vi "Read Spectrum.vi"(8 "error in (no error)":errorcluster, 11 "VISA resource name":refnum<visa-resource-name>) -> (0 "error out":errorcluster, 1 "Black Pixel Median":dbl, 2 "Spectrum by Pixel Number":dbl[](array[numeric]), 3 "VISA resource name out":refnum<visa-resource-name>)   [LabVIEW 2012, in "Ocean Optics 2000 4000.lvlib"]
doc: "Reads the optical or full spectra from the spectrometer, based on Pixel Mode selected in <b>Initalize</b> VI. The spectrum is displayed in an array according to the pixel number."
uses:
  Ocean Optics 2000 4000.lvlib
  <vilib>/Analysis/NI_AALBase.lvlib
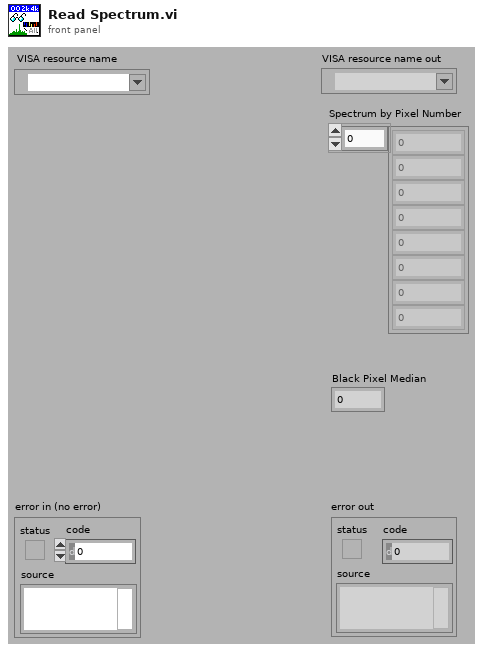
[diagram p1: front panel]
types:
  T1 = cluster{"Start Pixel":i32, "Stop Pixel":i32, "Start Black":i32[], "Stop Black":i32[]}
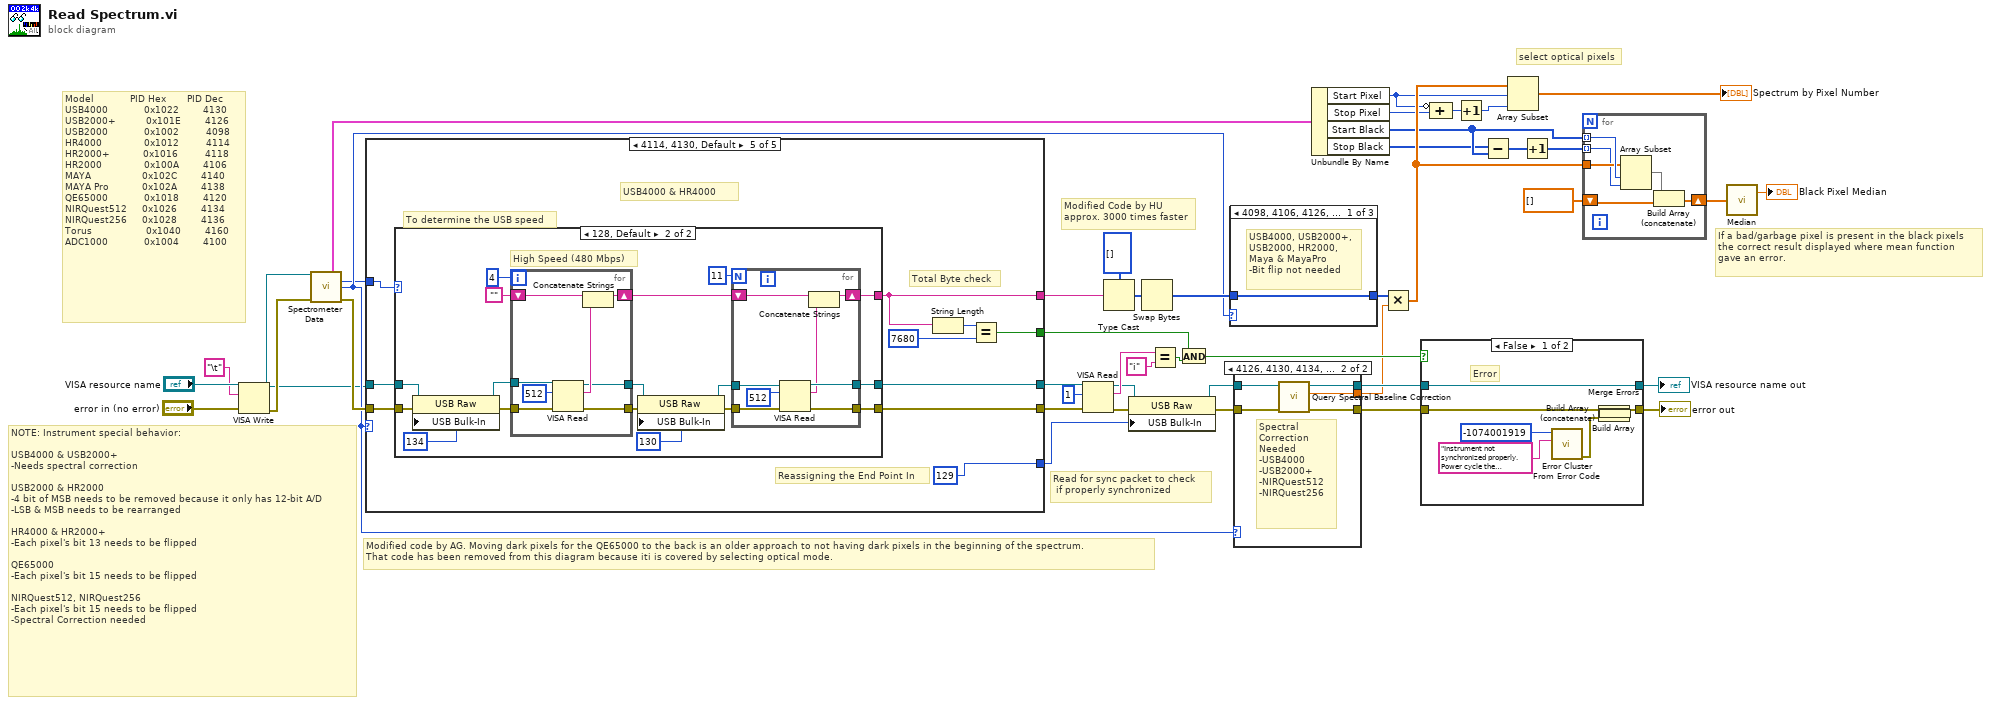
[diagram p0: block diagram]
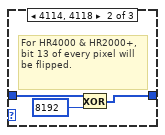
[diagram p2: hidden frame]
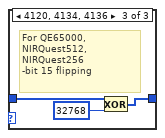
[diagram p3: hidden frame]
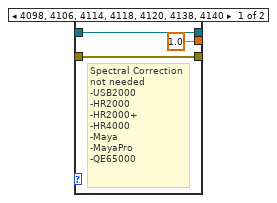
[diagram p4: hidden frame]
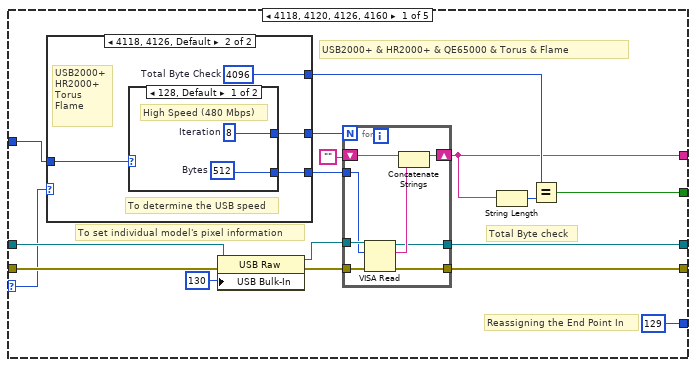
[diagram p5: hidden frame]
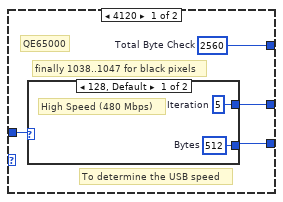
[diagram p6: hidden frame]
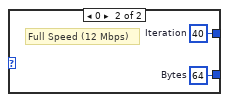
[diagram p7: hidden frame]
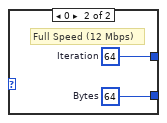
[diagram p8: hidden frame]
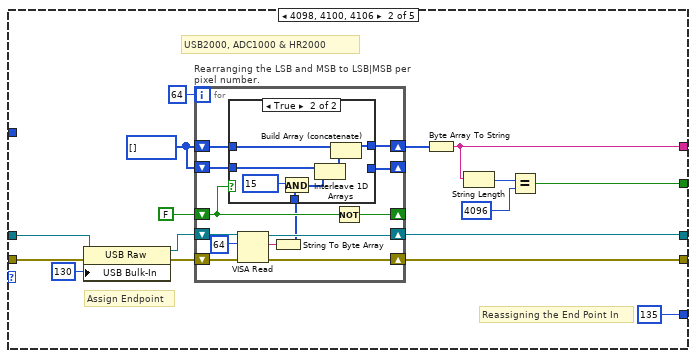
[diagram p9: hidden frame]
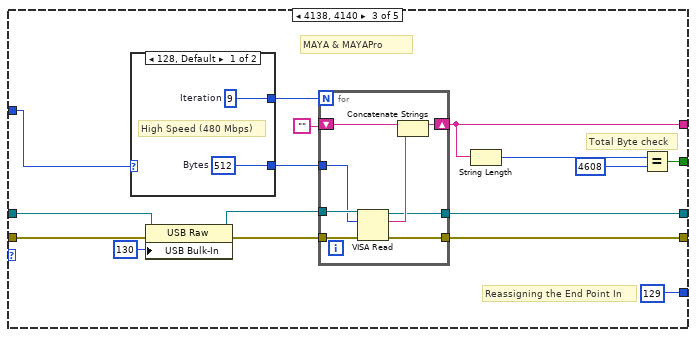
[diagram p11: hidden frame]
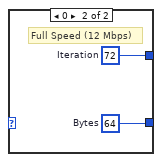
[diagram p12: hidden frame]
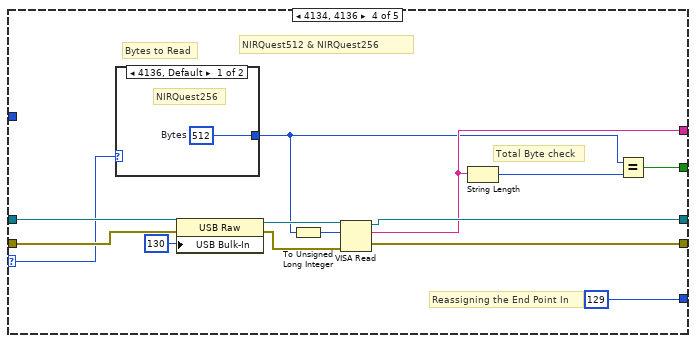
[diagram p13: hidden frame]
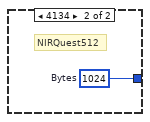
[diagram p14: hidden frame]
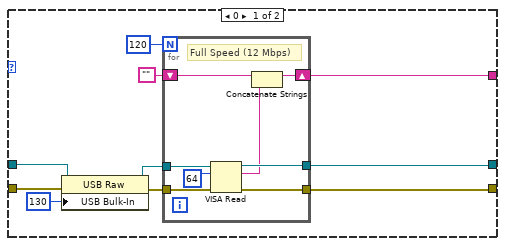
[diagram p15: hidden frame]
diagram:
  # "If a bad/garbage pixel is present in the black pixels\nthe correct result displayed where mean function\ngave an error."
  # "select optical pixels"
  # "Modified code by AG. Moving dark pixels for the QE65000 to the back is an older approach to not having dark pixels in the beginning of the spectrum.\nThat code has been removed from this diagram because iti is covered by selecting optical mode."
  # "Model            PID Hex       PID Dec \nUSB4000            0x1022        4130 \nUSB2000+          0x101E        4126 \nUSB2000            0x1002         4098\nHR4000              0x1012         4114\nHR2000+           0x1016         4118\nHR2000              0x100A        4106\nMAYA                 0x102C        4140\nMAYA Pro           0x102A        4138\nQE65000            0x1018        4120\nNIRQuest512     0x1026        4134\nNIRQuest256     0x1028        4136\nTorus                  0x1040        4160\nADC1000            0x1004        4100"
  # "Modified Code by HU\napprox. 3000 times faster"
  # "NOTE: Instrument special behavior:\n\nUSB4000 & USB2000+ \n-Needs spectral correction\n\nUSB2000 & HR2000\n-4 bit of MSB needs to be removed because it only has 12-bit A/D\n-LSB & MSB needs to be rearranged \n\nHR4000 & HR2000+\n-Each pixel's bit 13 needs to be flipped\n\nQE65000\n-Each pixel's bit 15 needs to be flipped\n\nNIRQuest512, NIRQuest256\n-Each pixel's bit 15 needs to be flipped \n-Spectral Correction needed"
  # "Read for sync packet to check\n if properly synchronized"
  n1 = VISA Write(VISA resource name="VISA resource name", write buffer="\t", error in (no error)="error in (no error)") -> (VISA resource name out=w2:refnum<visa-resource-name>, error out=w4:errorcluster)  [unwired: 1 out]
  n2 = call "Spectrometer Data.vi"("VISA resource name"=w2, "error in (no error)"=w4) -> ("Pixels"=w11:T1, "USB Speed"=w1:u16, "ID"=w3:u16, "error out"=w20:errorcluster)  [unwired: 8 in, 2 out]
  n3 = case shown="4114, 4130, Default" w3 {
    selector: w3 -> [w49 _ _ w161 _]
    tunnel: w2 -> [w61 w101 w140 w163 w178]
    tunnel: w20 -> [w62 w100 w139 w162 w177]
    tunnel: [w47 w89 w127 w156 w171] -> w27
    tunnel: [w60 w88 w138 w158 w176] -> w44
    tunnel: [w59 w87 w137 w157 w175] -> w43
    tunnel: [w58 w97 w134 w159 w173] -> w29
    tunnel: [i16 129 ("USB Settings:Bulk-In Pipe") i16 135 ("USB Settings:Bulk-In Pipe") i16 129 ("USB Settings:Bulk-In Pipe") i16 129 ("USB Settings:Bulk-In Pipe") i16 129 ("USB Settings:Bulk-In Pipe")] -> w28
    tunnel: w1 -> [w46 _ w125 _ w169]
    frame 4118, 4120, 4126, 4160 {
      # "To set individual model's pixel information"
      # "Total Byte check"
      # "Reassigning the End Point In"
      # "USB2000+ & HR2000+ & QE65000 & Torus & Flame"
      n4 = case shown="4118, 4126, Default" w49 {
        tunnel: w46 -> [w66 w74]
        tunnel: [w65 w73] -> w51
        tunnel: [w64 w72] -> w50
        tunnel: [w63 w71] -> w48
        frame 4120 {
          w63 = 2560  # Total Byte Check
          # "finally 1038..1047 for black pixels"
          # "To determine the USB speed"
          # "QE65000"
          n5 = case shown="128, Default" w66 {
            tunnel: [w68 w70] -> w65
            tunnel: [w67 w69] -> w64
            frame 128, Default {
              w67 = u32 512  # Bytes
              w68 = 5  # Iteration
              # "High Speed (480 Mbps)"
            }
            frame 0 {
              w69 = u32 64  # Bytes
              w70 = 40  # Iteration
              # "Full Speed (12 Mbps)"
            }
          }
        }
        frame 4118, 4126, Default {
          w71 = 4096  # Total Byte Check
          # "USB2000+ \nHR2000+\nTorus\nFlame"
          # "To determine the USB speed"
          n6 = case shown="128, Default" w74 {
            tunnel: [w76 w78] -> w73
            tunnel: [w75 w77] -> w72
            frame 128, Default {
              w75 = u32 512  # Bytes
              w76 = 8  # Iteration
              # "High Speed (480 Mbps)"
            }
            frame 0 {
              w77 = u32 64  # Bytes
              w78 = 64  # Iteration
              # "Full Speed (12 Mbps)"
            }
          }
        }
      }
      n7 = property class="USB Raw"(reference=w61, error in=w62, "USB Bulk-In"=i16 130 ("USB Settings:Bulk-In Pipe")) -> (reference out=w54:refnum<visa-resource-name>, error out=w53:errorcluster)
      n8 = for {
        N: w51 -> [_]
        tunnel: w54 -> [w86]
        tunnel: w53 -> [w85]
        shift-right: [w84] -> w47
        shift-left: "" -> [w83]
        tunnel: [w81] -> w60
        tunnel: [w80] -> w59
        tunnel: w50 -> [w79]
        n9 = VISA Read(VISA resource name=w86, byte count=w79, error in (no error)=w85) -> (VISA resource name out=w81:refnum<visa-resource-name>, read buffer=w82:string, error out=w80:errorcluster)  [unwired: 1 out]
        n10 = Concatenate Strings(w83, w82) -> (w84:string)
      }
      n11 = String Length(string=w47) -> (length=w57:i32)
      n12 = Equal?(x=w48, y=w57) -> (x = y?=w58:bool)
    }
    frame 4098, 4100, 4106 {
      w91 = u8[] []
      # "Reassigning the End Point In"
      # "Assign Endpoint"
      # "USB2000, ADC1000 & HR2000"
      n13 = property class="USB Raw"(reference=w101, error in=w100, "USB Bulk-In"=i16 130 ("USB Settings:Bulk-In Pipe")) -> (reference out=w94:refnum<visa-resource-name>, error out=w93:errorcluster)
      n14 = for "Rearranging the LSB and MSB to LSB|MSB per pixel number." {
        N: 64 -> [_]
        shift-right: [w115] -> _
        shift-left: FALSE -> [w114]
        shift-right: [w113] -> _
        shift-left: w91 -> [w112]
        shift-right: [w111] -> w90
        shift-left: w91 -> [w110]
        shift-right: [w105] -> w88
        shift-left: w94 -> [w108]
        shift-right: [w106] -> w87
        shift-left: w93 -> [w107]
        n15 = VISA Read(VISA resource name=w108, byte count=u32 64, error in (no error)=w107) -> (VISA resource name out=w105:refnum<visa-resource-name>, read buffer=w104:string, error out=w106:errorcluster)  [unwired: 1 out]
        n16 = String To Byte Array(string=w104) -> (unsigned byte array=w103:u8[])
        n17 = case shown="True" w114 {
          tunnel: [w116 _] -> w113
          tunnel: w112 -> [_ w124]
          tunnel: [w117 w120] -> w111
          tunnel: w110 -> [w117 w122]
          tunnel: w103 -> [w116 w118]
          frame False {
          }
          frame True {
            n18 = And(x=u8 15, y=w118) -> (x .and. y?=w121:u8[])
            n19 = Interleave 1D Arrays(w124, w121) -> (w123:u8[])
            n20 = Build Array (concatenate)(w122, w123) -> (w120:u8[])
          }
        }
        n21 = Not(x=w114) -> (.not. x?=w115:bool)
      }
      n22 = Byte Array To String(unsigned byte array=w90) -> (string=w89:string)
      n23 = String Length(string=w89) -> (length=w99:i32)
      n24 = Equal?(x=w99, y=4096) -> (x = y?=w97:bool)
    }
    frame 4138, 4140 {
      # "Reassigning the End Point In"
      # "Total Byte check"
      # "MAYA & MAYAPro"
      n25 = case shown="128, Default" w125 {
        tunnel: [w142 w144] -> w129
        tunnel: [w141 w143] -> w128
        frame 128, Default {
          w141 = u32 512  # Bytes
          w142 = 9  # Iteration
          # "High Speed (480 Mbps)"
        }
        frame 0 {
          w143 = u32 64  # Bytes
          w144 = 72  # Iteration
          # "Full Speed (12 Mbps)"
        }
      }
      n26 = property class="USB Raw"(reference=w140, error in=w139, "USB Bulk-In"=i16 130 ("USB Settings:Bulk-In Pipe")) -> (reference out=w132:refnum<visa-resource-name>, error out=w131:errorcluster)
      n27 = for {
        N: w129 -> [_]
        tunnel: w132 -> [w152]
        tunnel: w131 -> [w151]
        shift-right: [w150] -> w127
        shift-left: "" -> [w149]
        tunnel: [w147] -> w138
        tunnel: [w146] -> w137
        tunnel: w128 -> [w145]
        n28 = VISA Read(VISA resource name=w152, byte count=w145, error in (no error)=w151) -> (VISA resource name out=w147:refnum<visa-resource-name>, read buffer=w148:string, error out=w146:errorcluster)  [unwired: 1 out]
        n29 = Concatenate Strings(w149, w148) -> (w150:string)
      }
      n30 = String Length(string=w127) -> (length=w135:i32)
      n31 = Equal?(x=w135, y=4608) -> (x = y?=w134:bool)
    }
    frame 4134, 4136 {
      # "Reassigning the End Point In"
      # "Bytes to Read"
      # "Total Byte check"
      # "NIRQuest512 & NIRQuest256"
      n32 = case shown="4136, Default" w161 {
        tunnel: [w167 w168] -> w153
        frame 4136, Default {
          w167 = 512  # Bytes
          # "NIRQuest256"
        }
        frame 4134 {
          w168 = 1024  # Bytes
          # "NIRQuest512"
        }
      }
      n33 = property class="USB Raw"(reference=w163, error in=w162, "USB Bulk-In"=i16 130 ("USB Settings:Bulk-In Pipe")) -> (reference out=w165:refnum<visa-resource-name>, error out=w164:errorcluster)
      n34 = To Unsigned Long Integer(number=w153) -> (unsigned 32bit integer=w154:u32)
      n35 = VISA Read(VISA resource name=w165, byte count=w154, error in (no error)=w164) -> (VISA resource name out=w158:refnum<visa-resource-name>, read buffer=w156:string, error out=w157:errorcluster)  [unwired: 1 out]
      n36 = String Length(string=w156) -> (length=w160:i32)
      n37 = Equal?(x=w153, y=w160) -> (x = y?=w159:bool)
    }
    frame 4114, 4130, Default {
      # "Reassigning the End Point In"
      # "Total Byte check"
      # "To determine the USB speed"
      # "USB4000 & HR4000"
      n38 = case shown="128, Default" w169 {
        tunnel: w178 -> [w183 w213]
        tunnel: w177 -> [w182 w212]
        tunnel: [w181 w200] -> w176
        tunnel: [w180 w199] -> w175
        tunnel: [w179 w197] -> w171
        frame 0 {
          n39 = property class="USB Raw"(reference=w183, error in=w182, "USB Bulk-In"=i16 130 ("USB Settings:Bulk-In Pipe")) -> (reference out=w187:refnum<visa-resource-name>, error out=w184:errorcluster)
          n40 = for {
            N: 120 -> [_]
            tunnel: w187 -> [w195]
            tunnel: w184 -> [w194]
            tunnel: [w193] -> w181
            tunnel: [w192] -> w180
            shift-right: [w191] -> w179
            shift-left: "" -> [w190]
            # "Full Speed (12 Mbps)"
            n41 = VISA Read(VISA resource name=w195, byte count=u32 64, error in (no error)=w194) -> (VISA resource name out=w193:refnum<visa-resource-name>, read buffer=w189:string, error out=w192:errorcluster)  [unwired: 1 out]
            n42 = Concatenate Strings(w190, w189) -> (w191:string)
          }
        }
        frame 128, Default {
          # "High Speed (480 Mbps)"
          n43 = property class="USB Raw"(reference=w213, error in=w212, "USB Bulk-In"=i16 134 ("USB Settings:Bulk-In Pipe")) -> (reference out=w210:refnum<visa-resource-name>, error out=w209:errorcluster)
          n44 = for {
            N: 4 -> [_]
            tunnel: w210 -> [w221]
            tunnel: w209 -> [w220]
            shift-right: [w214] -> w198
            shift-left: "" -> [w218]
            tunnel: [w216] -> w204
            tunnel: [w215] -> w203
            n45 = VISA Read(VISA resource name=w221, byte count=u32 512, error in (no error)=w220) -> (VISA resource name out=w216:refnum<visa-resource-name>, read buffer=w217:string, error out=w215:errorcluster)  [unwired: 1 out]
            n46 = Concatenate Strings(w218, w217) -> (w214:string)
          }
          n47 = property class="USB Raw"(reference=w204, error in=w203, "USB Bulk-In"=i16 130 ("USB Settings:Bulk-In Pipe")) -> (reference out=w207:refnum<visa-resource-name>, error out=w201:errorcluster)
          n48 = for {
            N: 11 -> [_]
            tunnel: w207 -> [w228]
            tunnel: w201 -> [w227]
            tunnel: [w226] -> w200
            tunnel: [w225] -> w199
            shift-right: [w224] -> w197
            shift-left: w198 -> [w223]
            n49 = VISA Read(VISA resource name=w228, byte count=u32 512, error in (no error)=w227) -> (VISA resource name out=w226:refnum<visa-resource-name>, read buffer=w222:string, error out=w225:errorcluster)  [unwired: 1 out]
            n50 = Concatenate Strings(w223, w222) -> (w224:string)
          }
        }
      }
      n51 = String Length(string=w171) -> (length=w170:i32)
      n52 = Equal?(x=w170, y=7680) -> (x = y?=w173:bool)
    }
  }
  n53 = VISA Read(VISA resource name=w44, byte count=u32 1, error in (no error)=w43) -> (VISA resource name out=w38:refnum<visa-resource-name>, read buffer=w42:string, error out=w37:errorcluster)  [unwired: 1 out]
  n54 = Type Cast(type=u16[] [], x=w27) -> (*(type *) &x=w26:u16[])
  n55 = property class="USB Raw"(reference=w38, error in=w37, "USB Bulk-In"=w28) -> (reference out=w36:refnum<visa-resource-name>, error out=w35:errorcluster)
  n56 = Swap Bytes(anything=w26) -> (byte swapped=w24:u16[])
  n57 = Equal?(x=w42, y="i") -> (x = y?=w39:bool)
  n58 = And(x=w29, y=w39) -> (x .and. y?=w40:bool)
  n59 = case shown="4098, 4106, 4126, 4130, 4138, 4140, Default" w3 {
    tunnel: w24 -> [w230 w233 w235]
    tunnel: [w230 w231 w234] -> w23
    frame 4098, 4106, 4126, 4130, 4138, 4140, Default {
      # "USB4000, USB2000+, USB2000, HR2000, Maya & MayaPro\n-Bit flip not needed"
    }
    frame 4114, 4118 {
      # "For HR4000 & HR2000+, bit 13 of every pixel will be flipped."
      n60 = Exclusive Or(1:u16 8192 ("y"), 2:w233) -> (0:w231:u16[])
    }
    frame 4120, 4134, 4136 {
      # "For QE65000, NIRQuest512, NIRQuest256 \n-bit 15 flipping"
      n61 = Exclusive Or(1:u16 32768 ("y"), 2:w235) -> (0:w234:u16[])
    }
  }
  n62 = case shown="4126, 4130, 4134, 4136, Default" w3 {
    tunnel: w36 -> [w239 w244]
    tunnel: w35 -> [w238 w243]
    tunnel: [w239 w242] -> w34
    tunnel: [w238 w241] -> w33
    tunnel: [1.0 ("Spectral Baseline Correction") w240] -> w30
    frame 4098, 4106, 4114, 4118, 4120, 4138, 4140 {
      # "Spectral Correction not needed\n-USB2000\n-HR2000\n-HR2000+\n-HR4000\n-Maya\n-MayaPro\n-QE65000"
    }
    frame 4126, 4130, 4134, 4136, Default {
      # "Spectral Correction Needed\n-USB4000\n-USB2000+\n-NIRQuest512\n-NIRQuest256"
      n63 = call "Query Spectral Baseline Correction.vi"("error in (no error)"=w243, "VISA resource name"=w244) -> ("error out"=w241:errorcluster, "Spectral Baseline Correction"=w240:dbl, "VISA resource name out"=w242:refnum<visa-resource-name>)  [unwired: 7 out]
    }
  }
  n64 = Unbundle By Name(w11) -> ("Start Pixel"=w12:i32, "Stop Pixel"=w10:i32, "Start Black"=w9:i32[], "Stop Black"=w8:i32[])
  n65 = Multiply(x=w23, y=w30) -> (x*y=w22:dbl[])
  n66 = case shown="False" w40 {
    tunnel: w33 -> [w248 w254]
    tunnel: [w250 w254] -> w31
    tunnel: [w249 w253] -> w32
    tunnel: w34 -> [w249 w253]
    frame False {
      # "Error"
      n67 = call <vilib>:"Error Cluster From Error Code.vi"("error message (\"\")"="Instrument not synchronized properly. Power cycle the instrument." ("error message (\"\")"), "error code (0)"=-1074001919 ("code")) -> ("error out"=w247:errorcluster)  [unwired: 2 in, 5 out]
      n68 = Build Array(w248, w247) -> (w246:errorcluster[])
      n69 = Build Array (concatenate)(w246) -> (w245:errorcluster[])
      n70 = Merge Errors(w245) -> (w250:errorcluster)
    }
    frame True {
      # "No error. Instrument properly synchronized."
    }
  }
  "VISA resource name out" <- w32
  "error out" <- w31
  n71 = Compound Arithmetic op=ADD(invert w12, w10) -> (w17:i32)
  n72 = Increment(x=w17) -> (x+1=w16:i32)
  n73 = Subtract(x=w8, y=w9) -> (x-y=w19:i32[])
  n74 = Array Subset(array=w22, index=w12, length=w16) -> (→"Spectrum by Pixel Number":dbl[])
  n75 = Increment(x=w19) -> (x+1=w18:i32[])
  n76 = for {
    tunnel: w9 -> [w260] mode=indexing
    tunnel: w22 -> [w259]
    tunnel: w18 -> [w258] mode=indexing
    shift-right: [w256] -> w14
    shift-left: dbl[] [] -> [w255]
    n77 = Array Subset(array=w259, index=w260, length=w258) -> (w257:dbl[])
    n78 = Build Array (concatenate)(w257, w255) -> (w256:dbl[])
  }
  n79 = call <vilib>:"Median.vi"("X"=w14) -> ("median"=→"Black Pixel Median":dbl)  [unwired: 1 out]
